vi "Actor Create.vi"(9 "Nested Alias":string, 10 "Nested Actor":refnum<class "Actor.lvclass">, 11 "Dev Actor in":refnum<class "Dev Actor.lvclass">) -> (3 "Dev Actor out":refnum<class "Dev Actor.lvclass">)   [LabVIEW 2021, in "Dev Actor.lvlib" / "Dev Actor.lvclass"]
uses:
  Dev Actor.lvclass
  <vilib>/jettl/jettl/jettl/Actor/Actor.lvclass
  Dev Actor.lvclass/Dev Actor.ctl
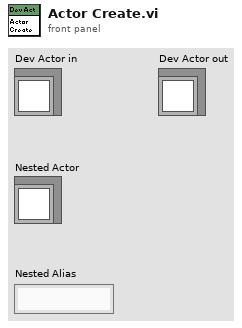
[diagram p1: front panel]
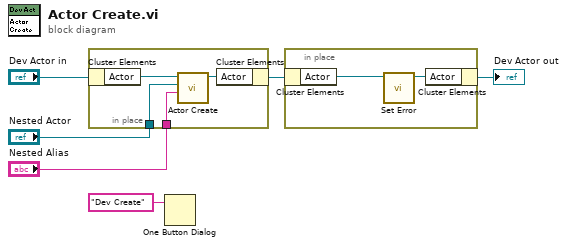
[diagram p0: block diagram]
diagram:
  n1 = in-place {
    in-place-border: "Nested Actor" -> [w8]
    in-place-border: "Nested Alias" -> [w7]
    n2 = in-place-cluster #1("Dev Actor in") -> ("Actor"=w10:refnum<class "Actor.lvclass">)
    n3 = call-dynamic "Actor Create.vi"("Nested Alias"=w7, "Nested Actor"=w8, "Actor Create in"=w10) -> ("Actor Create out"=w9:refnum<class "Actor.lvclass">)  [unwired: 8 in]
    n4 = in-place-cluster #1("Actor"=w9) -> (w4:refnum<class "Dev Actor.lvclass">)
  }
  n5 = One Button Dialog(message="Dev Create") -> ()  [unwired: 1 in, 1 out]
  n6 = in-place {
    n7 = in-place-cluster #2(w4) -> ("Actor"=w12:refnum<class "Actor.lvclass">)
    n8 = call-dynamic "Set Error.vi"("Actor in"=w12) -> ("Actor out"=w11:refnum<class "Actor.lvclass">)  [unwired: 10 in]
    n9 = in-place-cluster #2("Actor"=w11) -> (→"Dev Actor out":refnum<class "Dev Actor.lvclass">)
  }
